vi "Clase String's.vi"() -> ()   [LabVIEW 2018]
panel:
  out "result string":string
  in  "Ocultar":bool
  out "Tab Control":enum32{"Login", "Admin", "Users", "Welcome"}(tab)
  in  "Pass":string
  in  "Loggin":bool
  in  "User":string
  out "Directory":string
  out "Aclaración":string
  in  "Users":bool
  in  "Delete":bool
  in  "Username":string
  in  "Password":string
  in  "Add":bool
  in  "Loggout":bool
  in  "Loggout 2":bool
  out "Sesión iniciada por:":string
  out "Usuarios dados de alta:":string[][](array[string])
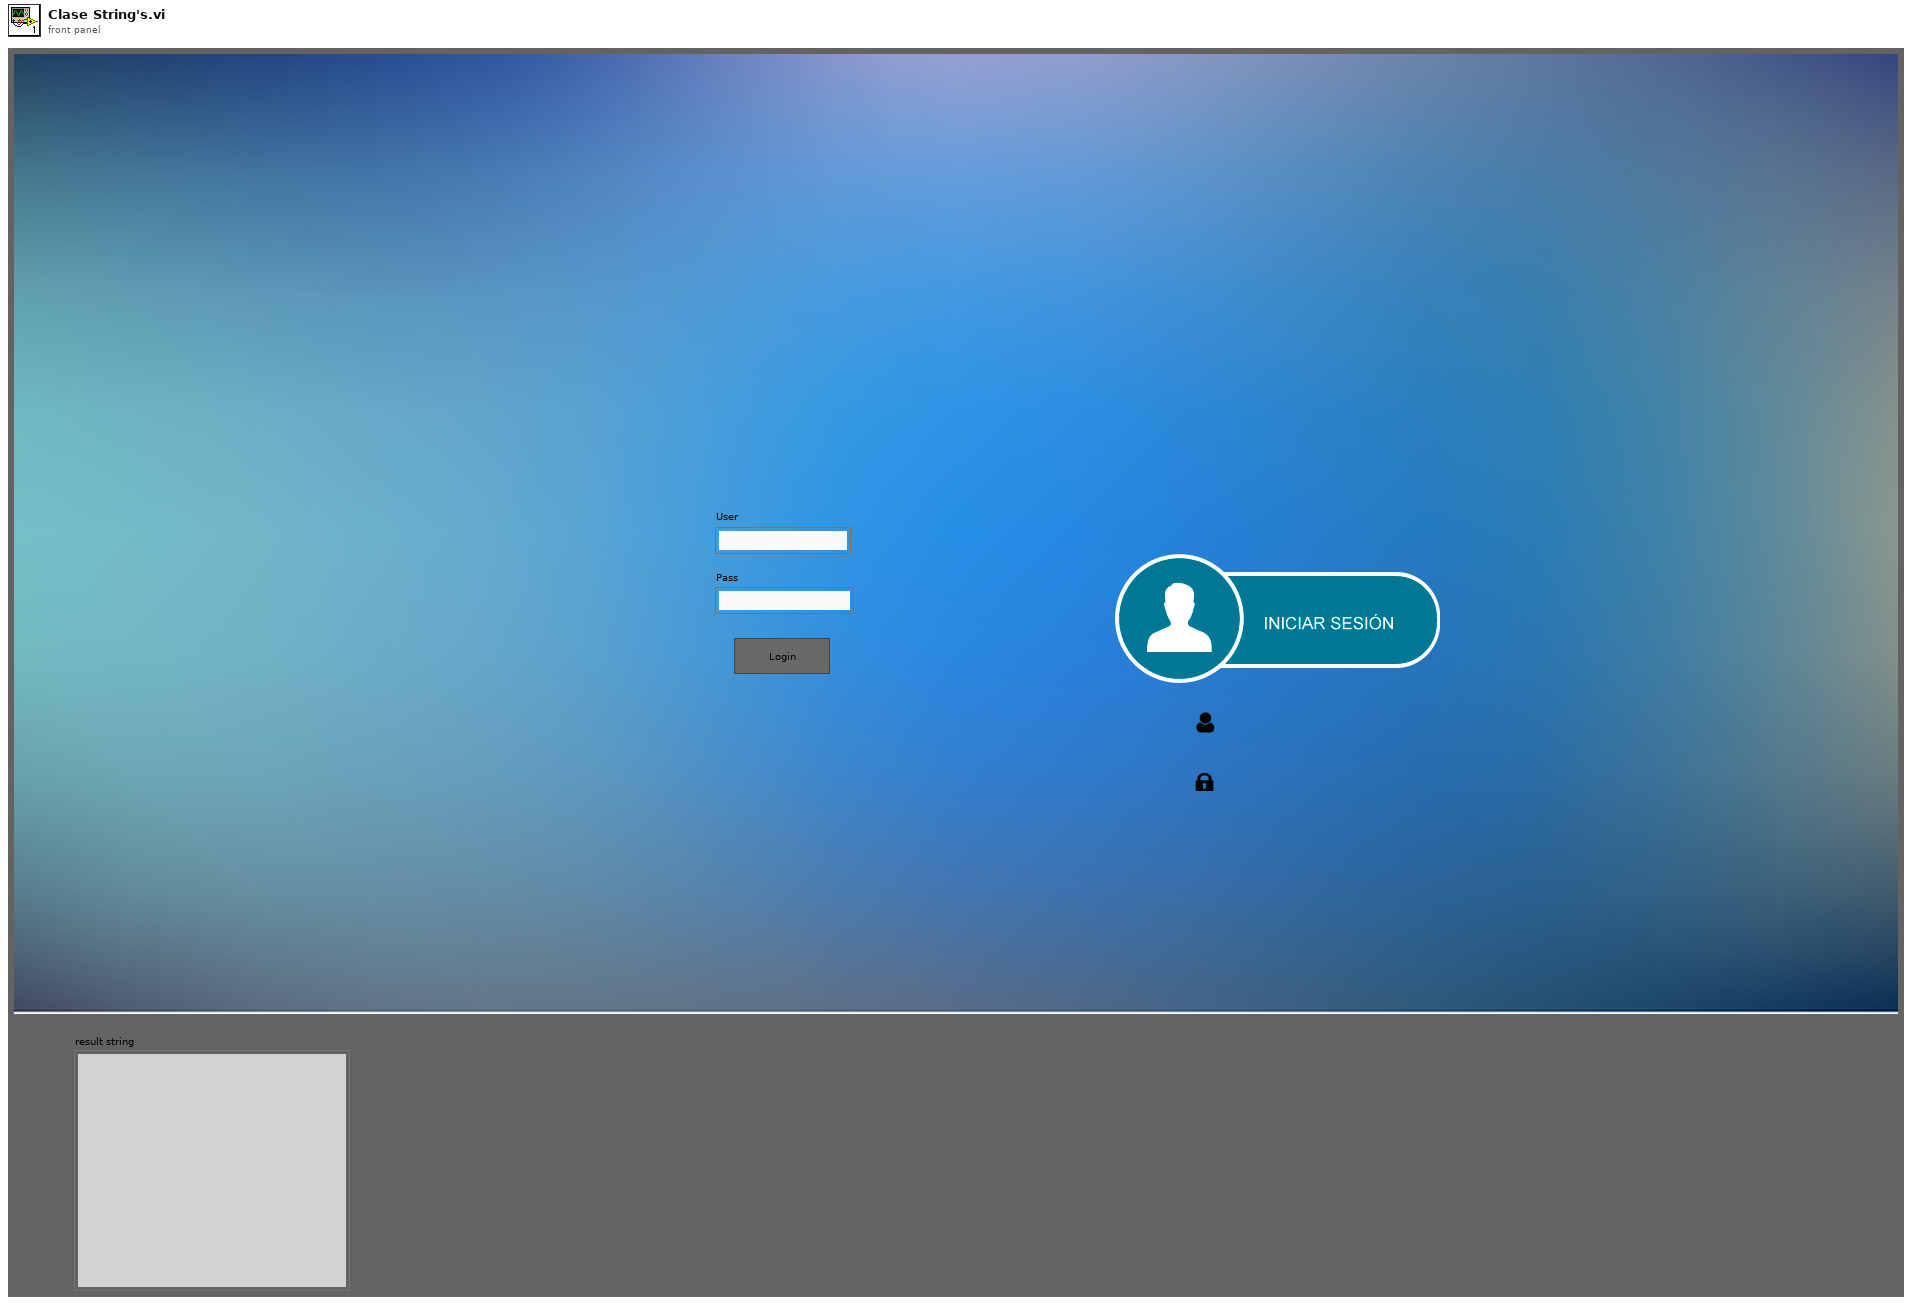
[diagram p1: front panel]
types:
  T1 = enum16{"open", "replace", "create", "open or create", "replace or create", "replace or create with confirmation"}
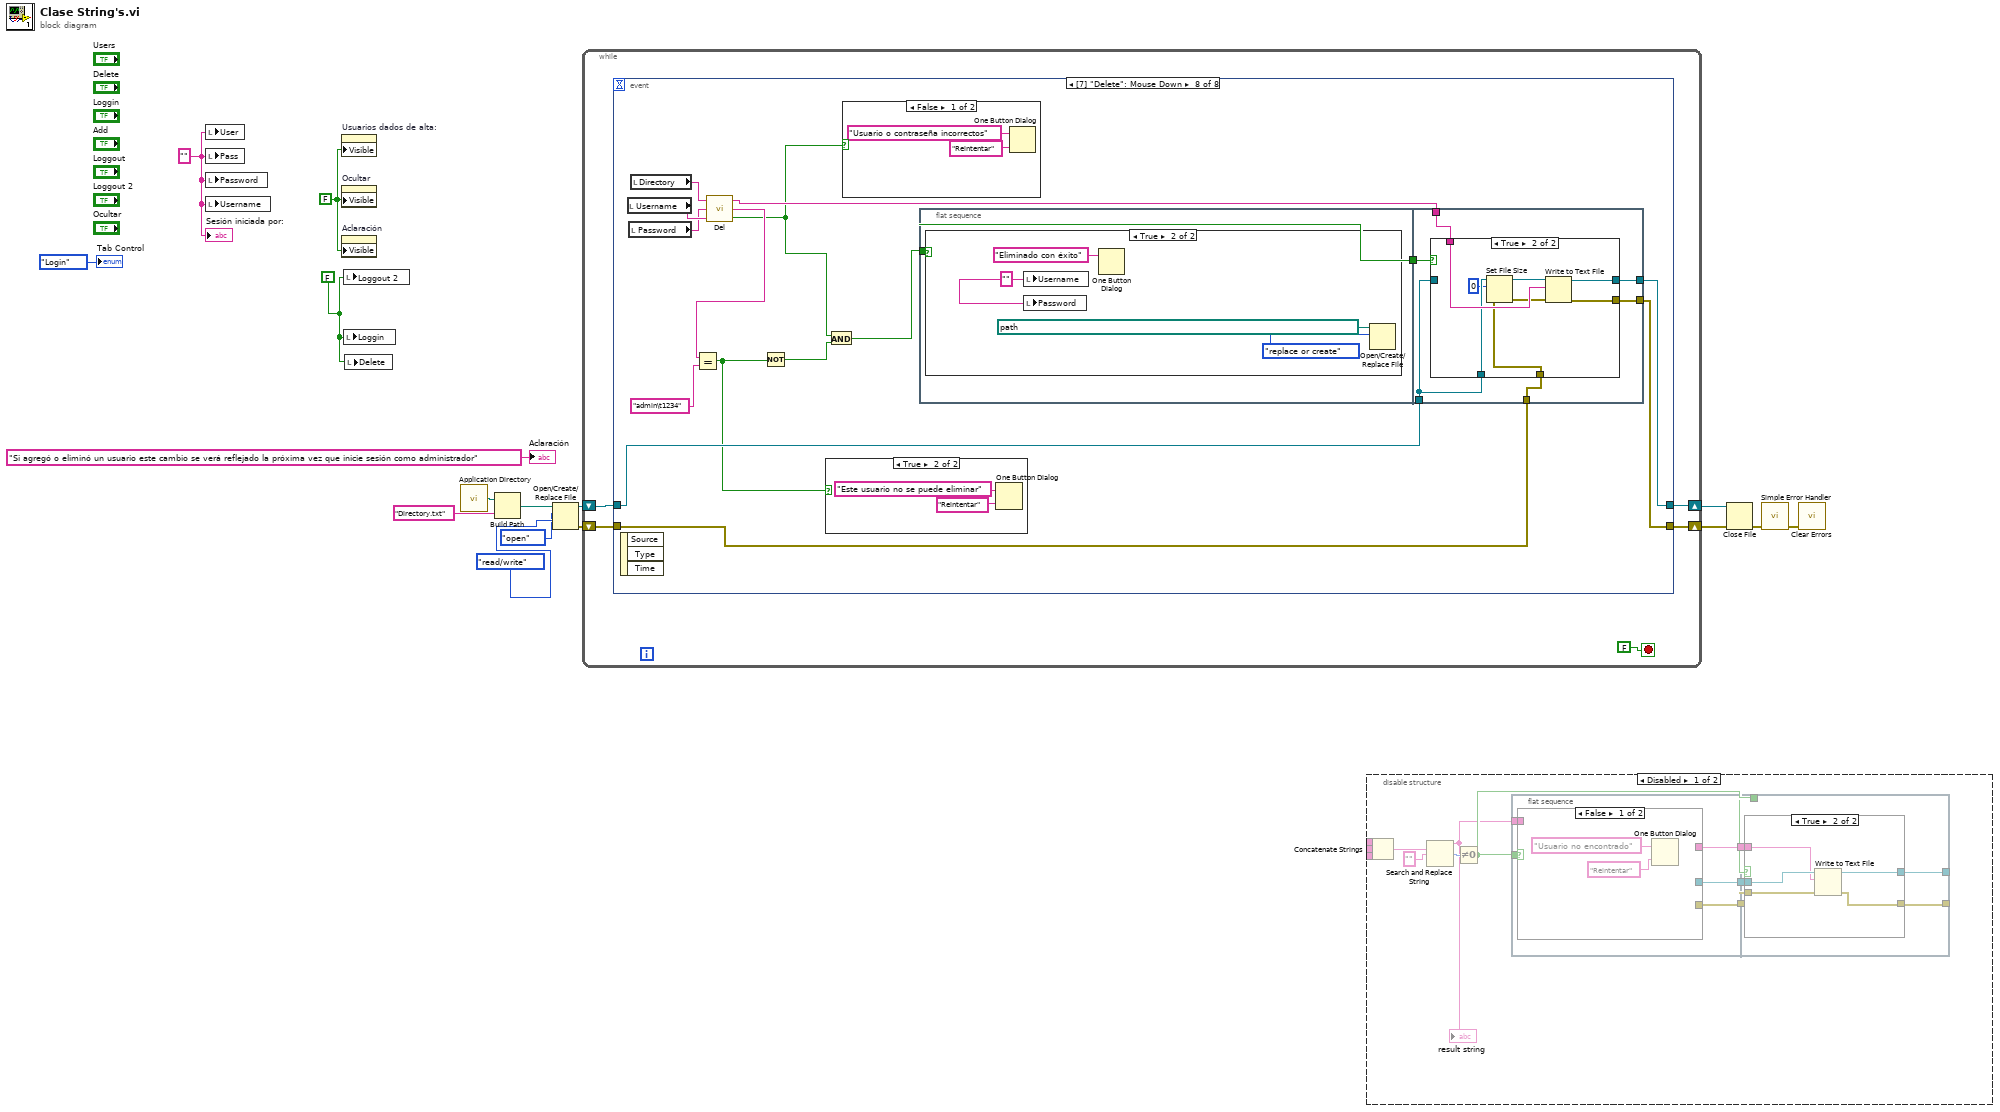
[diagram p0: block diagram]
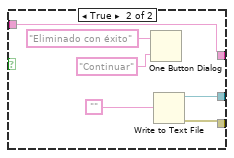
[diagram p2: hidden frame]
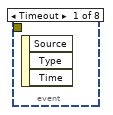
[diagram p5: hidden frame]
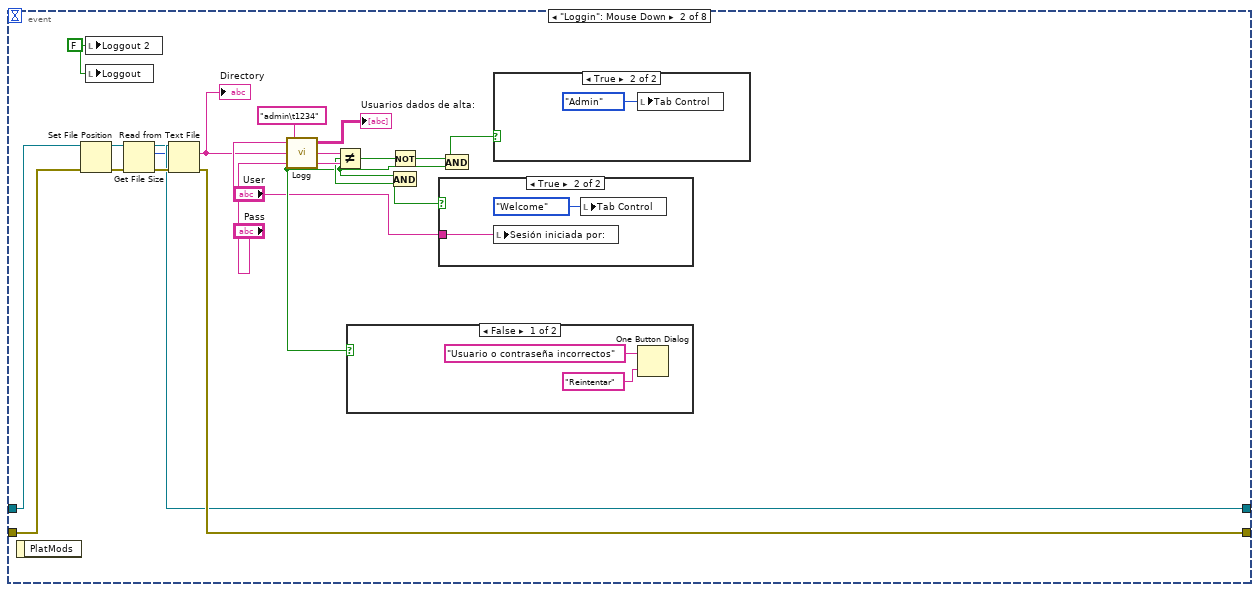
[diagram p6: hidden frame]
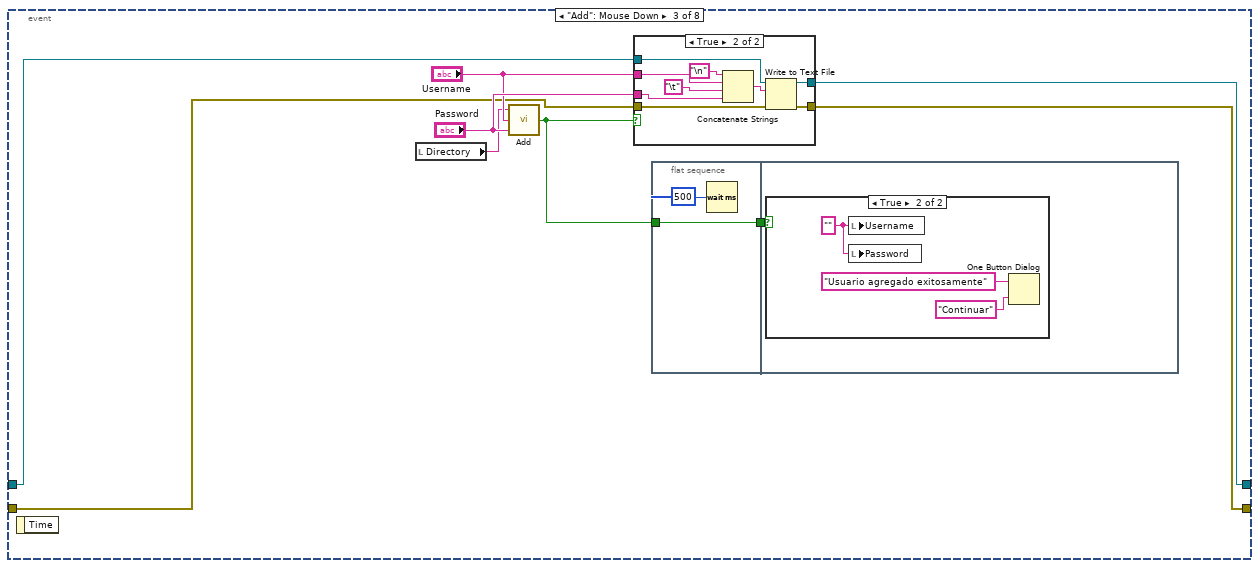
[diagram p10: hidden frame]
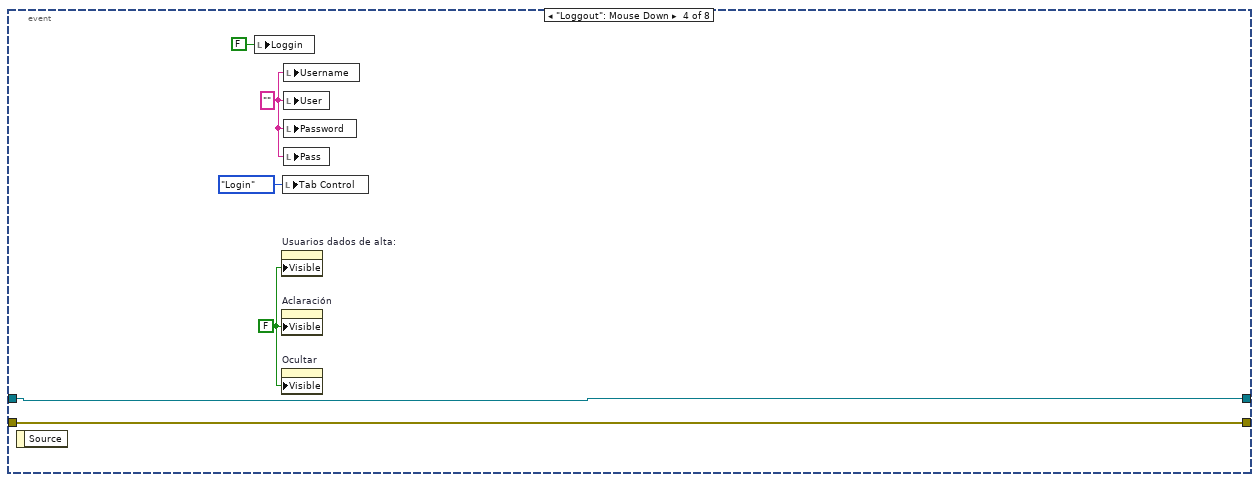
[diagram p13: hidden frame]
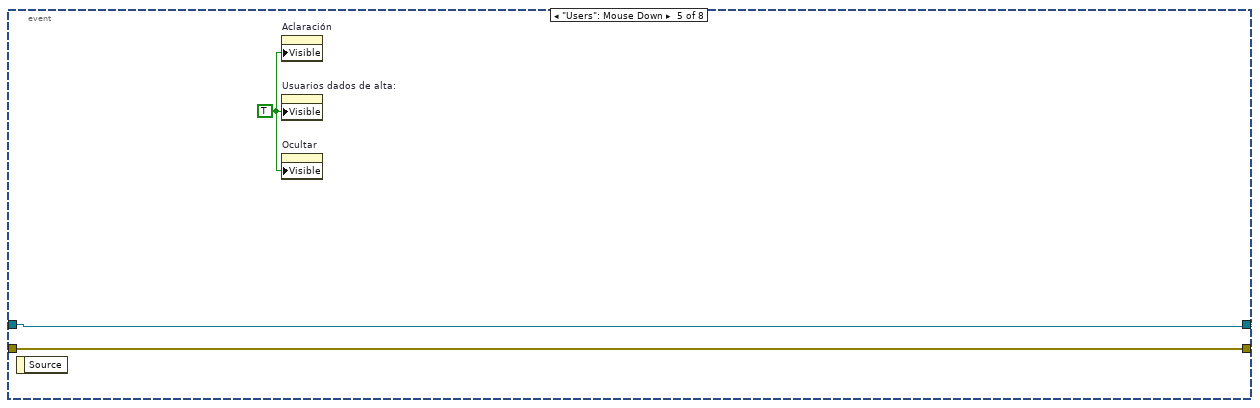
[diagram p14: hidden frame]
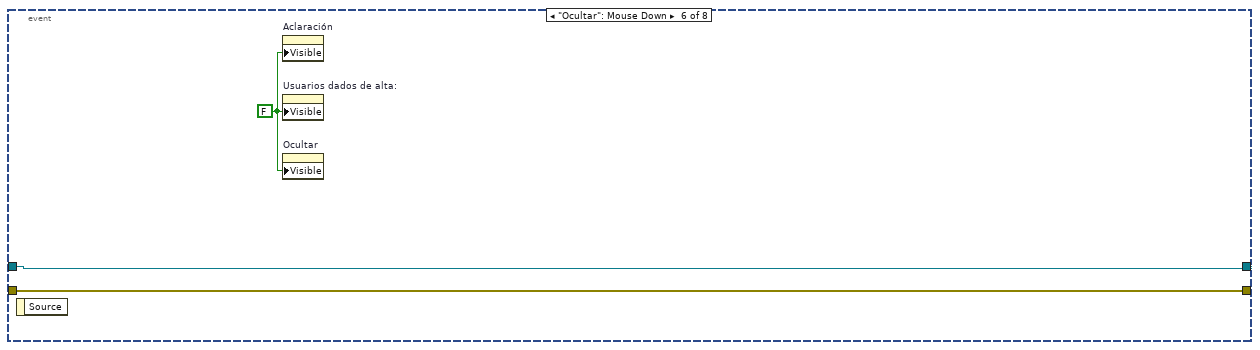
[diagram p15: hidden frame]
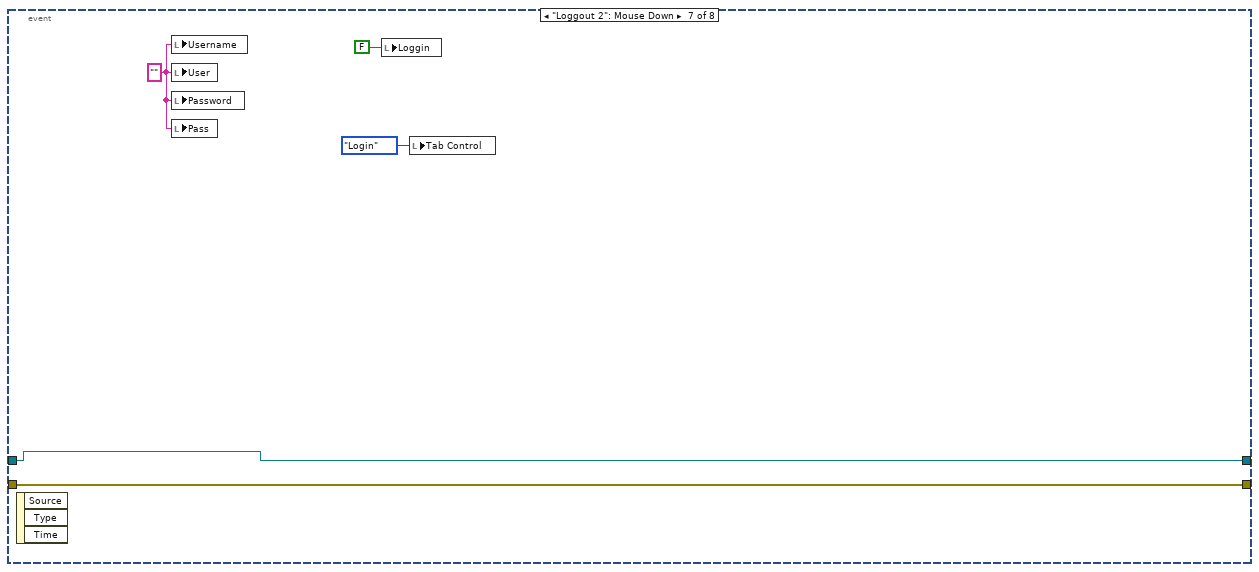
[diagram p16: hidden frame]
diagram:
  w3 = FALSE ("Visible")
  w1 = FALSE ("OK Button")
  w2 = "" ("User")
  n1 = local write "User"(w2) -> ()
  n2 = local write "Pass"(w2) -> ()
  n3 = local write "Password"(w2) -> ()
  n4 = local write "Username"(w2) -> ()
  n5 = property on="Usuarios dados de alta:" class="Arr (strict)"("Visible"=w3) -> ()  [unwired: 2 in, 2 out]
  n6 = property on="Ocultar" class="Bool (strict)"("Visible"=w3) -> ()  [unwired: 2 in, 2 out]
  n7 = property on="Aclaración" class="Str"("Visible"=w3) -> ()  [unwired: 2 in, 2 out]
  n8 = local write "Loggout 2"(w1) -> ()
  n9 = local write "Loggin"(w1) -> ()
  n10 = local write "Delete"(w1) -> ()
  n11 = call <vilib>:"Application Directory.vi"() -> ("Application Directory"=w16:path)
  n12 = Build Path(base path=w16, name or relative path="Directory.txt") -> (appended path=w15:path)
  n13 = Open/Create/Replace File(file path (use dialog)=w15, operation (0:open)=T1."open", access (0:read/write)=enum16{"read/write", "read-only", "write-only"}."read/write") -> (refnum out=w12:refnum<file>, error out=w11:errorcluster)  [unwired: 3 in, 1 out]
  n14 = while {
    shift-right: [w20] -> w6
    shift-left: w11 -> [w18]
    shift-right: [w19] -> w10
    shift-left: w12 -> [w17]
    stop <- FALSE stop-if-true
    n15 = event shown="[7] \"Delete\": Mouse Down" {
      selector: _ -> [_ _ _ _ _ _ _ _]
      dyn-events: _ -> [_ _ _ _ _ _ _ _]
      timeout: _ -> [_ _ _ _ _ _ _ _]
      tunnel: [_ w40 w52 w75 w81 w84 w85 w102] -> w20
      tunnel: [_ w38 w51 w73 w79 w82 w86 w103] -> w19
      tunnel: w18 -> [_ w39 w53 w75 w81 w84 w85 w91]
      tunnel: w17 -> [_ w27 w48 w73 w79 w82 w86 w104]
      event Timeout {
        n16 = event-data() -> ()  [unwired: 1 in, 3 out]
      }
      event "Loggin": Mouse Down {
        w28 = FALSE ("OK Button")
        n17 = event-data() -> ()  [unwired: 1 in, 1 out]
        n18 = Set File Position(refnum=w27, error in=w39) -> (refnum out=w36:refnum<file>, error out=w42:errorcluster)  [unwired: 2 in]
        n19 = local write "Loggout 2"(w28) -> ()
        n20 = local write "Loggout"(w28) -> ()
        n21 = Get File Size(file=w36, error in=w42) -> (refnum out=w37:refnum<file>, size (in bytes)=w35:i64, 0:w41:errorcluster)
        n22 = Read from Text File(file (use dialog)=w37, count=w35, error in=w41) -> (refnum out=w38:refnum<file>, text=w23:string, error out=w40:errorcluster)  [unwired: 1 in, 1 out]
        "Directory" <- w23
        n23 = call "Logg.vi"("Pass"="Pass", "Datos"=w23, "User"="User") -> ("Logg"=w25:bool, "Usuario"=w26:string, "Usuarios"=→"Usuarios dados de alta:":string[][])
        n24 = Not Equal?(x=w26, y="admin\t1234") -> (x != y?=w33:bool)
        n25 = case shown="False" w25 {
          frame False {
            n26 = One Button Dialog(message="Usuario o contraseña incorrectos", button name ("OK")="Reintentar") -> ()  [unwired: 1 out]
          }
          frame True {
          }
        }
        n27 = Not(x=w33) -> (.not. x?=w32:bool)
        n28 = And(x=w25, y=w33) -> (x .and. y?=w30:bool)
        n29 = case shown="True" w30 {
          tunnel: "User" -> [_ w47]
          frame False {
          }
          frame True {
            n30 = local write "Sesión iniciada por:"(w47) -> ()
            n31 = local write "Tab Control"(enum32{"Login", "Admin", "Users", "Welcome"}."Welcome" ("Tab Control")) -> ()
          }
        }
        n32 = And(x=w32, y=w25) -> (x .and. y?=w31:bool)
        n33 = case shown="True" w31 {
          frame False {
          }
          frame True {
            n34 = local write "Tab Control"(enum32{"Login", "Admin", "Users", "Welcome"}."Admin" ("Tab Control")) -> ()
          }
        }
      }
      event "Add": Mouse Down {
        n35 = event-data() -> ()  [unwired: 1 in, 1 out]
        n36 = local read "Directory"() -> (w50:string)
        n37 = call "Add.vi"("Password"="Password", "Username"="Username", "Datos"=w50) -> ("Added"=w56:bool)
        n38 = case shown="True" w56 {
          tunnel: "Username" -> [_ w70]
          tunnel: "Password" -> [_ w69]
          tunnel: [_ w68] -> w51
          tunnel: [w63 w67] -> w52
          tunnel: w53 -> [w63 w66]
          tunnel: w48 -> [_ w64]
          frame False {
          }
          frame True {
            n39 = Concatenate Strings("\n", w70, "\t", w69) -> (w72:string)
            n40 = Write to Text File(file (use dialog)=w64, text=w72, error in=w66) -> (refnum out=w68:refnum<file>, error out=w67:errorcluster)  [unwired: 1 in, 1 out]
          }
        }
        n41 = flat-sequence {
          tunnel: w56 -> [w58]
          tunnel: [w58] -> w49
          tunnel: w49 -> [w59]
          frame #0 {
            n42 = Wait (ms)(milliseconds to wait=u32 500) -> ()  [unwired: 1 out]
          }
          frame #1 {
            n43 = case shown="True" w59 {
              frame False {
              }
              frame True {
                w60 = "" ("Username")
                n44 = local write "Username"(w60) -> ()
                n45 = local write "Password"(w60) -> ()
                n46 = One Button Dialog(message="Usuario agregado exitosamente", button name ("OK")="Continuar") -> ()  [unwired: 1 out]
              }
            }
          }
        }
      }
      event "Loggout": Mouse Down {
        w74 = FALSE ("Visible")
        w77 = "" ("User")
        n47 = event-data() -> ()  [unwired: 1 in, 1 out]
        n48 = local write "Loggin"(FALSE ("OK Button")) -> ()
        n49 = property on="Usuarios dados de alta:" class="Arr (strict)"("Visible"=w74) -> ()  [unwired: 2 in, 2 out]
        n50 = property on="Aclaración" class="Str"("Visible"=w74) -> ()  [unwired: 2 in, 2 out]
        n51 = property on="Ocultar" class="Bool (strict)"("Visible"=w74) -> ()  [unwired: 2 in, 2 out]
        n52 = local write "Tab Control"(enum32{"Login", "Admin", "Users", "Welcome"}."Login" ("Tab Control")) -> ()
        n53 = local write "Username"(w77) -> ()
        n54 = local write "User"(w77) -> ()
        n55 = local write "Password"(w77) -> ()
        n56 = local write "Pass"(w77) -> ()
      }
      event "Users": Mouse Down {
        w80 = TRUE ("Visible")
        n57 = event-data() -> ()  [unwired: 1 in, 1 out]
        n58 = property on="Aclaración" class="Str"("Visible"=w80) -> ()  [unwired: 2 in, 2 out]
        n59 = property on="Usuarios dados de alta:" class="Arr (strict)"("Visible"=w80) -> ()  [unwired: 2 in, 2 out]
        n60 = property on="Ocultar" class="Bool (strict)"("Visible"=w80) -> ()  [unwired: 2 in, 2 out]
      }
      event "Ocultar": Mouse Down {
        w83 = FALSE ("Visible")
        n61 = event-data() -> ()  [unwired: 1 in, 1 out]
        n62 = property on="Aclaración" class="Str"("Visible"=w83) -> ()  [unwired: 2 in, 2 out]
        n63 = property on="Usuarios dados de alta:" class="Arr (strict)"("Visible"=w83) -> ()  [unwired: 2 in, 2 out]
        n64 = property on="Ocultar" class="Bool (strict)"("Visible"=w83) -> ()  [unwired: 2 in, 2 out]
      }
      event "Loggout 2": Mouse Down {
        w88 = "" ("User")
        n65 = event-data() -> ()  [unwired: 1 in, 3 out]
        n66 = local write "Username"(w88) -> ()
        n67 = local write "User"(w88) -> ()
        n68 = local write "Password"(w88) -> ()
        n69 = local write "Pass"(w88) -> ()
        n70 = local write "Loggin"(FALSE ("OK Button")) -> ()
        n71 = local write "Tab Control"(enum32{"Login", "Admin", "Users", "Welcome"}."Login" ("Tab Control")) -> ()
      }
      event "Delete": Mouse Down {
        n72 = event-data() -> ()  [unwired: 1 in, 3 out]
        n73 = local read "Username"() -> (w95:string)
        n74 = local read "Password"() -> (w94:string)
        n75 = local read "Directory"() -> (w96:string)
        n76 = call "Del.vi"("User"=w95, "Pass"=w94, "Datos"=w96) -> ("Del OK?"=w90:bool, "Usuario"=w92:string, "Directorio Nuevo"=w93:string)
        n77 = Equal?(x=w92, y="admin\t1234") -> (x = y?=w100:bool)
        n78 = Not(x=w100) -> (.not. x?=w99:bool)
        n79 = case shown="True" w100 {
          frame False {
          }
          frame True {
            n80 = One Button Dialog(message="Este usuario no se puede eliminar", button name ("OK")="Reintentar") -> ()  [unwired: 1 out]
          }
        }
        n81 = And(x=w90, y=w99) -> (x .and. y?=w98:bool)
        n82 = case shown="False" w90 {
          frame False {
            n83 = One Button Dialog(message="Usuario o contraseña incorrectos", button name ("OK")="Reintentar") -> ()  [unwired: 1 out]
          }
          frame True {
          }
        }
        n84 = flat-sequence {
          tunnel: [w109] -> w97
          tunnel: w98 -> [w109]
          tunnel: w104 -> [w114]
          tunnel: [w119] -> w103
          tunnel: [w118] -> w102
          tunnel: w97 -> [w117]
          tunnel: w93 -> [w116]
          tunnel: w91 -> [w115]
          frame #0 {
            n85 = case shown="True" w109 {
              frame False {
              }
              frame True {
                w110 = "" ("Username")
                n86 = local write "Username"(w110) -> ()
                n87 = local write "Password"(w110) -> ()
                n88 = One Button Dialog(message="Eliminado con éxito") -> ()  [unwired: 1 in, 1 out]
                n89 = Open/Create/Replace File(file path (use dialog)=path "C:/Users/Diego/Documents/Universidad/Programación II/Quiz 3/Directory.txt", operation (0:open)=T1."replace or create") -> ()  [unwired: 4 in, 3 out]
              }
            }
          }
          frame #1 {
            n90 = case shown="True" w117 {
              tunnel: w114 -> [w120 _]
              tunnel: [w120 w128] -> w119
              tunnel: [_ w127] -> w118
              tunnel: w116 -> [_ w125]
              tunnel: w115 -> [_ w123]
              tunnel: w114 -> [_ w122]
              frame False {
              }
              frame True {
                n91 = Set File Size(4:w123, 6:i64 0 ("size (in bytes)"), 7:w122) -> (0:w124:errorcluster, 3:w126:refnum<file>)
                n92 = Write to Text File(file (use dialog)=w126, text=w125, error in=w124) -> (refnum out=w128:refnum<file>, error out=w127:errorcluster)  [unwired: 1 in, 1 out]
              }
            }
          }
        }
      }
    }
  }
  n93 = disable-structure shown="Disabled" {
    disable-tunnel: _ -> [w135 _]
    disable-tunnel: _ -> [w134 _]
    disable-tunnel: _ -> [w133 _]
    frame Disabled {
      n94 = Concatenate Strings(w134, w135, w133) -> (w132:string)
      n95 = Search and Replace String(search string=w132, replace string="" ("search string")) -> (result string=w129:string, number of replacements=w131:i32)  [unwired: 6 in, 2 out]
      "result string" <- w129
      n96 = Not Equal To 0?(x=w131) -> (x != 0?=w130:bool)
      n97 = flat-sequence {
        tunnel: w130 -> [w144]
        tunnel: [w143] -> w139
        tunnel: [w142] -> w138
        tunnel: w129 -> [w141]
        tunnel: [w140] -> w137
        tunnel: [w157] -> _
        tunnel: w139 -> [w158]
        tunnel: w130 -> [w156]
        tunnel: [w155] -> _
        tunnel: w138 -> [w154]
        tunnel: w137 -> [w153]
        frame #0 {
          n98 = case shown="False" w144 {
            tunnel: [_ w150] -> w143
            tunnel: [_ w149] -> w142
            tunnel: [_ w148] -> w140
            tunnel: w141 -> [_ w148]
            frame False {
              n99 = One Button Dialog(message="Usuario no encontrado", button name ("OK")="Reintentar") -> ()  [unwired: 1 out]
            }
            frame True {
              n100 = One Button Dialog(message="Eliminado con éxito", button name ("OK")="Continuar") -> ()  [unwired: 1 out]
              n101 = Write to Text File(text="") -> (refnum out=w149:refnum<file>, error out=w150:errorcluster)  [unwired: 3 in, 1 out]
            }
          }
        }
        frame #1 {
          n102 = case shown="True" w156 {
            tunnel: w158 -> [w159 w164]
            tunnel: [w159 w163] -> w157
            tunnel: [_ w162] -> w155
            tunnel: w154 -> [_ w161]
            tunnel: w153 -> [_ w160]
            frame False {
            }
            frame True {
              n103 = Write to Text File(file (use dialog)=w161, text=w160, error in=w164) -> (refnum out=w162:refnum<file>, error out=w163:errorcluster)  [unwired: 1 in, 1 out]
            }
          }
        }
      }
    }
    frame Enabled {
    }
  }
  n104 = Close File(refnum=w10, error in=w6) -> (error out=w7:errorcluster)  [unwired: 1 out]
  n105 = call <vilib>:"Simple Error Handler.vi"("error in (no error)"=w7) -> ("error out"=w5:errorcluster)  [unwired: 4 in, 4 out]
  n106 = call <vilib>:"Clear Errors.vi"("error in (no error)"=w5) -> ()  [unwired: 5 in, 2 out]
  "Tab Control" <- enum32{"Login", "Admin", "Users", "Welcome"}."Login" ("Tab Control")
  "Sesión iniciada por:" <- w2
  "Aclaración" <- "Si agregó o eliminó un usuario este cambio se verá reflejado la próxima vez que inicie sesión como administrador" ("Aclaración")
